vi "Problem 14.vi"(11 "Start Number":u64=999999) -> (3 "Answer":u64)   [LabVIEW 2013, in "Problem 14.lvlib"]
uses:
  Problem 14.lvlib
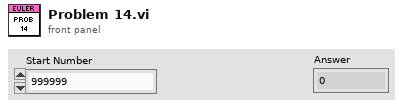
[diagram p1: front panel]
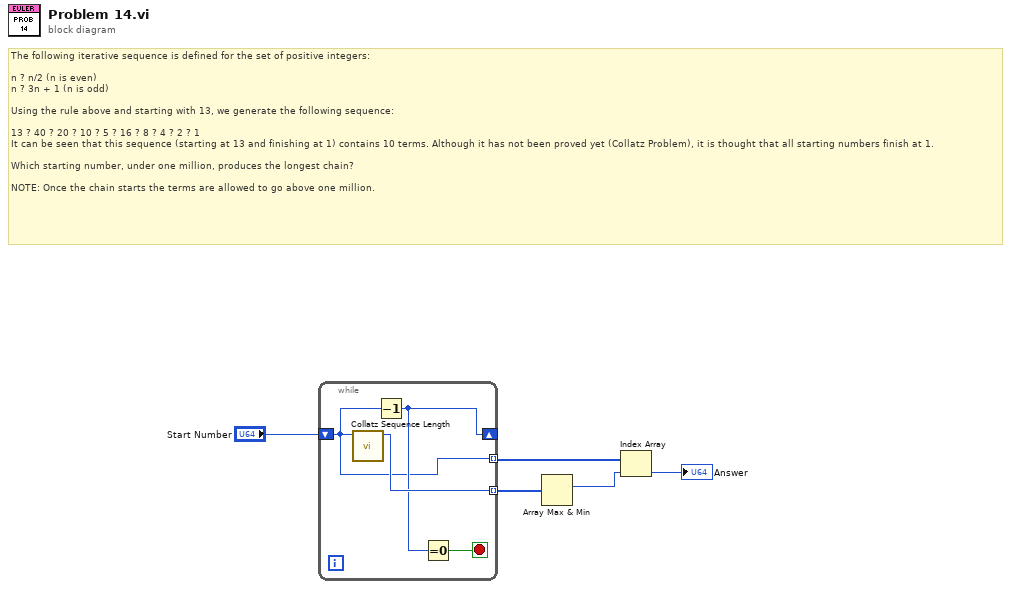
[diagram p0: block diagram]
diagram:
  # "The following iterative sequence is defined for the set of positive integers:\n\nn ? n/2 (n is even)\nn ? 3n + 1 (n is odd)\n\nUsing the rule above and starting with 13, we generate the following sequence:\n\n13 ? 40 ? 20 ? 10 ? 5 ? 16 ? 8 ? 4 ? 2 ? 1\nIt can be seen that this sequence (starting at 13 and finishing at 1) contains 10 terms. Although it has not been proved yet (Collatz Problem), it is thought that all starting numbers finish at 1.\n\nWhich starting number, under one million, produces the longest chain?\n\nNOTE: Once the chain starts the terms are allowed to go above one million."
  n1 = while {
    tunnel: [w9] -> w4 mode=indexing
    shift-right: [w7] -> _
    shift-left: "Start Number" -> [w6]
    tunnel: [w6] -> w3 mode=indexing
    stop <- w8 stop-if-true
    n2 = call "Collatz Sequence Length.vi"("n"=w6) -> ("Sequence Length"=w9:i32)  [unwired: 10 in]
    n3 = Decrement(x=w6) -> (x-1=w7:u64)
    n4 = Equal To 0?(x=w7) -> (x = 0?=w8:bool)
  }
  n5 = Array Max & Min(array=w4) -> (max index (indices)=w2:i32)  [unwired: 3 out]
  n6 = Index Array(array=w3, index=w2) -> (element=→"Answer":u64)
